vi "HXG2_PGLY-Props_R2.vi"(8 "error in (no error)":errorcluster, 9 "Temp Flowmeter (°F)":dbl, 10 "Rho PGLY Sensor(lbm/ft³)":dbl, 11 "PGLY Avg (°F)":dbl) -> (0 "error out":errorcluster, 1 "Concent":dbl, 2 "mu (lbm/ft*s)":dbl, 3 "Cp (BTU/lbm°F)":dbl, 4 "Density (lbm/ft³)":dbl)   [LabVIEW 2012]
uses:
  <vilib>/gmath/NI_Gmath.lvlib
panel:
  out "appended array":dbl[](array[numeric])
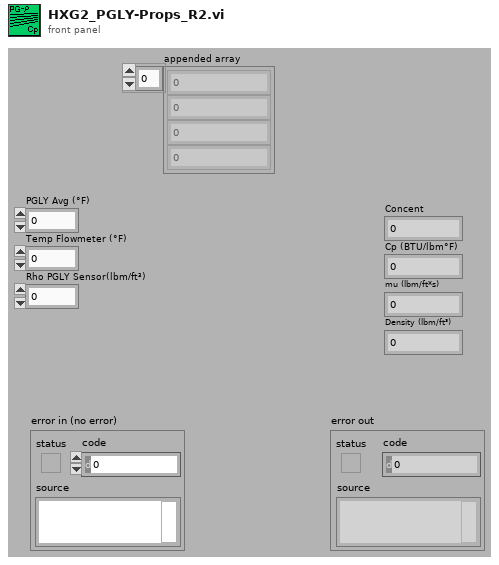
[diagram p1: front panel]
types:
  T1 = cluster{"[0]":dbl, "[1]":dbl, "[2]":dbl, "[3]":dbl}
  T2 = cluster{"[0]":dbl, "[1]":dbl, "[2]":dbl, "[3]":dbl, "[4]":dbl, "[5]":dbl, "[6]":dbl}
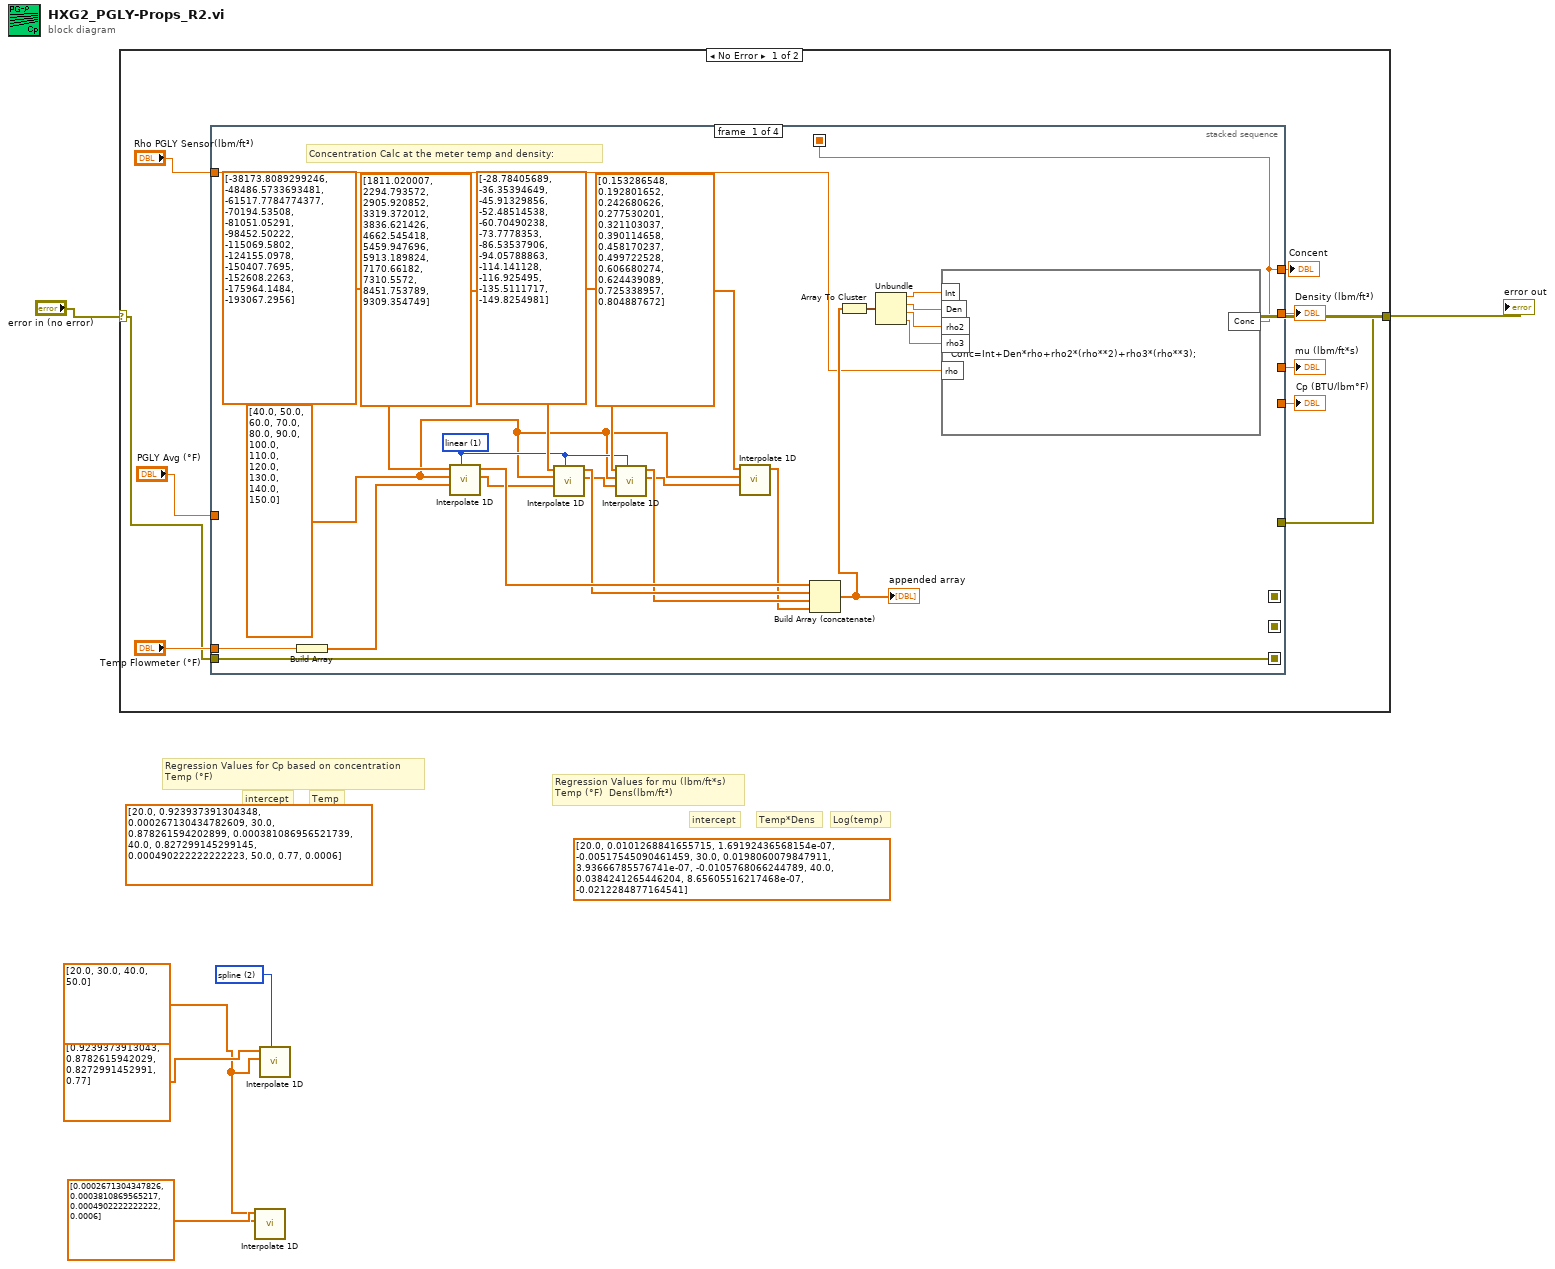
[diagram p0: block diagram]
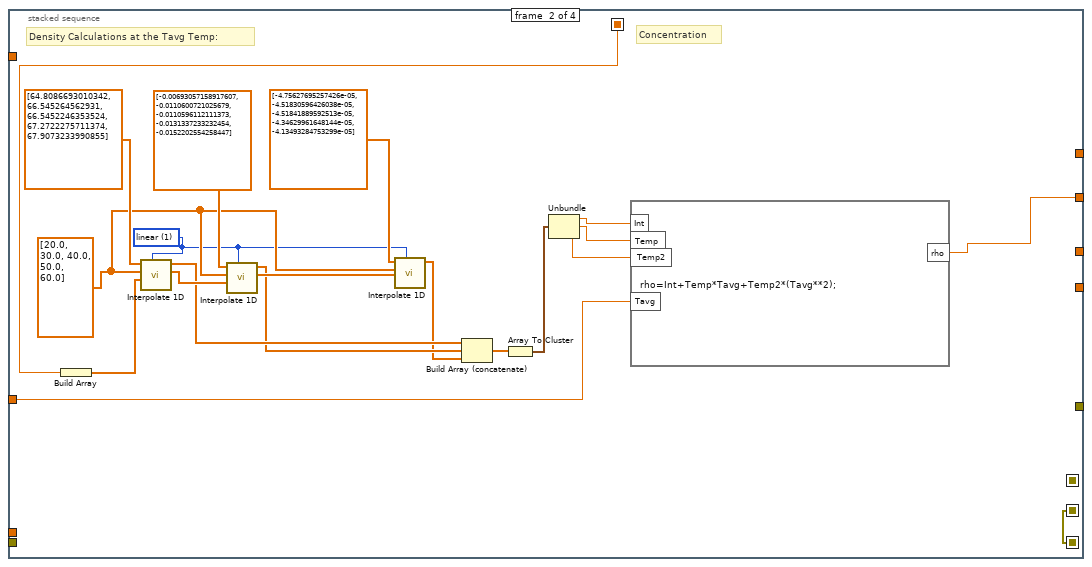
[diagram p2: hidden frame]
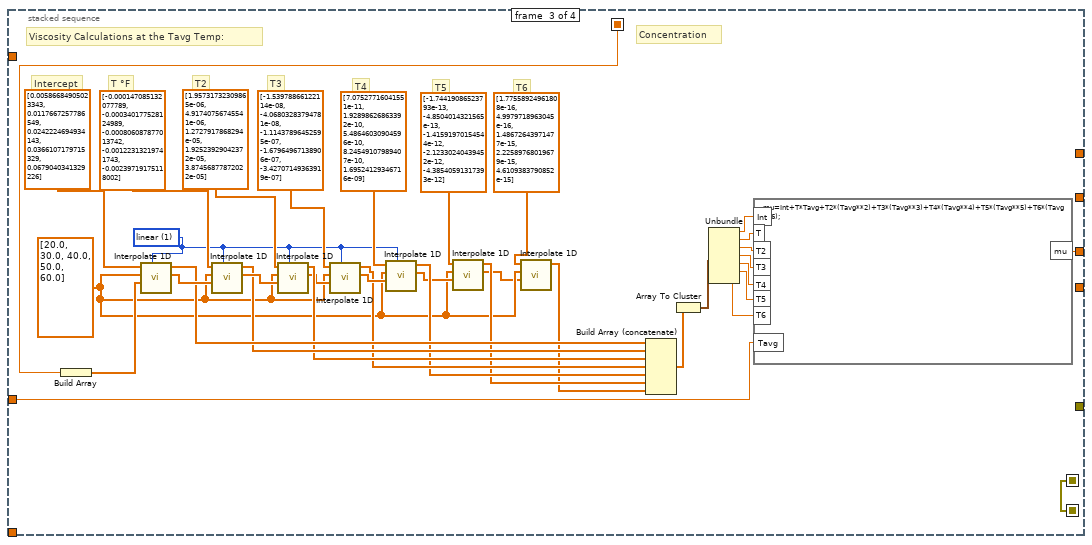
[diagram p3: hidden frame]
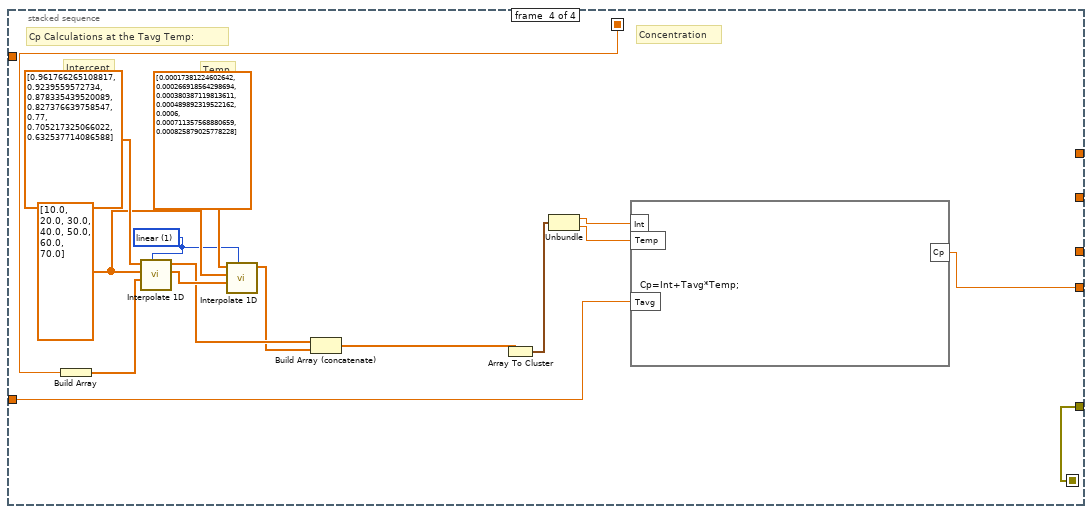
[diagram p4: hidden frame]
diagram:
  (unwired) dbl[][] [[20.0, 0.0101268841655715, 1.69192436568154e-07, -0.00517545090461459], [30.0, 0.0198060079847911, 3.93666785576741e-07, -0.0105768066244789], [40.0, 0.0384241265446204, 8.65605516217468e-07, -0.0212284877164541]]
  w4 = 2 items=["nearest", "linear", "spline", "cubic Hermite", "Lagrange"] ("method")
  w1 = dbl[] [20.0, 30.0, 40.0, 50.0] ("array")
  (unwired) dbl[][] [[20.0, 0.923937391304348, 0.000267130434782609], [30.0, 0.878261594202899, 0.000381086956521739], [40.0, 0.827299145299145, 0.000490222222222223], [50.0, 0.77, 0.0006]] ("array")
  # "Temp"
  # "intercept"
  # "Log(temp)"
  # "Temp*Dens"
  # "intercept"
  # "Regression Values for mu (lbm/ft*s)\nTemp (°F)  Dens(lbm/ft³)"
  # "Regression Values for Cp based on concentration\nTemp (°F)"
  n1 = case shown="No Error" "error in (no error)" {
    selector: "error in (no error)" -> [w12 w112]
    tunnel: [w7 w112] -> w5
    frame No Error {
      n2 = stacked-sequence {
        seq-local: [w17 _ _ _] -> [_ w43 _ _]
        seq-local: [w16 _ _ _] -> [_ w42 w82 w100]
        seq-local: [_ w43 _ _] -> [_ _ w79 _]
        seq-local: [_ _ w79 _] -> [_ _ _ w96]
        tunnel: "Temp Flowmeter (°F)" -> [w19 _ _ _]
        tunnel: "Rho PGLY Sensor(lbm/ft³)" -> [w18 _ _ _]
        tunnel: [w16 _ _ _] -> w13
        tunnel: w12 -> [w17 _ _ _]
        tunnel: [_ w44 _ _] -> w11
        tunnel: "PGLY Avg (°F)" -> [_ w40 w80 w98]
        tunnel: [_ _ w78 _] -> w9
        tunnel: [_ _ _ w97] -> w8
        tunnel: [_ _ _ w96] -> w7
        frame #0 {
          w31 = 1 items=["nearest", "linear", "spline", "cubic Hermite", "Lagrange"] ("method")
          w27 = dbl[] [40.0, 50.0, 60.0, 70.0, 80.0, 90.0, 100.0, 110.0, 120.0, 130.0, 140.0, 150.0]
          # "Concentration Calc at the meter temp and density:"
          n3 = Build Array(w19) -> (w38:dbl[])
          n4 = call <vilib>:"Interpolate 1D.vi"("method"=w31, "xi"=w38, "X"=w27, "Y"=dbl[] [-38173.8089299246, -48486.5733693481, -61517.7784774377, -70194.53508, -81051.05291, -98452.50222, -115069.5802, -124155.0978, -150407.7695, -152608.2263, -175964.1484, -193067.2956]) -> ("xi used"=w35:dbl[], "yi"=w37:dbl[])  [unwired: 5 in, 1 out]
          n5 = call <vilib>:"Interpolate 1D.vi"("method"=w31, "xi"=w35, "X"=w27, "Y"=dbl[] [1811.020007, 2294.793572, 2905.920852, 3319.372012, 3836.621426, 4662.545418, 5459.947696, 5913.189824, 7170.66182, 7310.5572, 8451.753789, 9309.354749]) -> ("xi used"=w33:dbl[], "yi"=w34:dbl[])  [unwired: 5 in, 1 out]
          n6 = call <vilib>:"Interpolate 1D.vi"("method"=w31, "xi"=w33, "X"=w27, "Y"=dbl[] [-28.78405689, -36.35394649, -45.91329856, -52.48514538, -60.70490238, -73.7778353, -86.53537906, -94.05788863, -114.141128, -116.925495, -135.5111717, -149.8254981]) -> ("xi used"=w29:dbl[], "yi"=w30:dbl[])  [unwired: 5 in, 1 out]
          n7 = call <vilib>:"Interpolate 1D.vi"("xi"=w29, "X"=w27, "Y"=dbl[] [0.153286548, 0.192801652, 0.242680626, 0.277530201, 0.321103037, 0.390114658, 0.458170237, 0.499722528, 0.606680274, 0.624439089, 0.725338957, 0.804887672]) -> ("yi"=w26:dbl[])  [unwired: 6 in, 2 out]
          n8 = Build Array (concatenate)(w37, w34, w30, w26) -> (w25:dbl[])
          "appended array" <- w25
          n9 = Array To Cluster(array=w25) -> (cluster=w24:T1)
          n10 = Unbundle(w24) -> ("[0]"=w23:dbl, "[1]"=w22:dbl, "[2]"=w21:dbl, "[3]"=w20:dbl)
          n11 = formula code="Conc=Int+Den*rho+rho2*(rho**2)+rho3*(rho**3);"("Int"=w23, "Den"=w22, "rho2"=w21, "rho3"=w20, "rho"=w18) -> ("Conc"=w16:dbl)
        }
        frame #1 {
          w53 = 1 items=["nearest", "linear", "spline", "cubic Hermite", "Lagrange"] ("method")
          w54 = dbl[] [20.0, 30.0, 40.0, 50.0, 60.0]
          # "Density Calculations at the Tavg Temp:"
          # "Concentration"
          n12 = Build Array(w42) -> (w41:dbl[])
          n13 = call <vilib>:"Interpolate 1D.vi"("method"=w53, "xi"=w41, "X"=w54, "Y"=dbl[] [64.8086693010342, 66.545264562931, 66.5452246353524, 67.2722275711374, 67.9073233990855]) -> ("xi used"=w58:dbl[], "yi"=w52:dbl[])  [unwired: 5 in, 1 out]
          n14 = call <vilib>:"Interpolate 1D.vi"("method"=w53, "xi"=w58, "X"=w54, "Y"=dbl[] [-0.00693057158917607, -0.0110600721025679, -0.0110596112111373, -0.0131337233232454, -0.0152202554258447]) -> ("xi used"=w55:dbl[], "yi"=w51:dbl[])  [unwired: 5 in, 1 out]
          n15 = call <vilib>:"Interpolate 1D.vi"("method"=w53, "xi"=w55, "X"=w54, "Y"=dbl[] [-4.75627695257426e-05, -4.51830596426038e-05, -4.51841889592513e-05, -4.34629961648144e-05, -4.13493284753299e-05]) -> ("yi"=w50:dbl[])  [unwired: 5 in, 2 out]
          n16 = Build Array (concatenate)(w52, w51, w50) -> (w49:dbl[])
          n17 = Array To Cluster(array=w49) -> (cluster=w48:cluster{"[0]":dbl, "[1]":dbl, "[2]":dbl})
          n18 = Unbundle(w48) -> ("[0]"=w47:dbl, "[1]"=w46:dbl, "[2]"=w45:dbl)
          n19 = formula code="rho=Int+Temp*Tavg+Temp2*(Tavg**2);"("Int"=w47, "Temp"=w46, "Temp2"=w45, "Tavg"=w40) -> ("rho"=w44:dbl)
        }
        frame #2 {
          w72 = 1 items=["nearest", "linear", "spline", "cubic Hermite", "Lagrange"] ("method")
          w62 = dbl[] [20.0, 30.0, 40.0, 50.0, 60.0]
          # "T6"
          # "T5"
          # "T4"
          # "T3"
          # "T2"
          # "T °F"
          # "Intercept"
          # "Viscosity Calculations at the Tavg Temp:"
          # "Concentration"
          n20 = Build Array(w82) -> (w81:dbl[])
          n21 = call <vilib>:"Interpolate 1D.vi"("method"=w72, "xi"=w81, "X"=w62, "Y"=dbl[] [0.00586684905023343, 0.0117667257786549, 0.0242224694934143, 0.0366107179715329, 0.0679040341329226]) -> ("xi used"=w94:dbl[], "yi"=w90:dbl[])  [unwired: 5 in, 1 out]
          n22 = call <vilib>:"Interpolate 1D.vi"("method"=w72, "xi"=w94, "X"=w62, "Y"=dbl[] [-0.000147085132077789, -0.000340177528124989, -0.000806087877013742, -0.00122313219741743, -0.00239719175118002]) -> ("xi used"=w91:dbl[], "yi"=w89:dbl[])  [unwired: 5 in, 1 out]
          n23 = call <vilib>:"Interpolate 1D.vi"("method"=w72, "xi"=w91, "X"=w62, "Y"=dbl[] [1.95731732309865e-06, 4.91740756745541e-06, 1.2727917868294e-05, 1.92523929042372e-05, 3.87456877872022e-05]) -> ("xi used"=w77:dbl[], "yi"=w88:dbl[])  [unwired: 5 in, 1 out]
          n24 = call <vilib>:"Interpolate 1D.vi"("method"=w72, "xi"=w77, "X"=w62, "Y"=dbl[] [-1.53978866122114e-08, -4.06803283794781e-08, -1.11437896452595e-07, -1.67964967138906e-07, -3.42707149363919e-07]) -> ("xi used"=w74:dbl[], "yi"=w73:dbl[])  [unwired: 5 in, 1 out]
          n25 = call <vilib>:"Interpolate 1D.vi"("method"=w72, "xi"=w74, "X"=w62, "Y"=dbl[] [7.07527716041551e-11, 1.92898626863392e-10, 5.48646030904596e-10, 8.24549107989407e-10, 1.69524129346716e-09]) -> ("xi used"=w68:dbl[], "yi"=w69:dbl[])  [unwired: 5 in, 1 out]
          n26 = call <vilib>:"Interpolate 1D.vi"("xi"=w68, "X"=w62, "Y"=dbl[] [-1.74419086523793e-13, -4.8504014321565e-13, -1.41591970154544e-12, -2.12330240439452e-12, -4.38540591317393e-12]) -> ("xi used"=w60:dbl[], "yi"=w67:dbl[])  [unwired: 6 in, 1 out]
          n27 = call <vilib>:"Interpolate 1D.vi"("xi"=w60, "X"=w62, "Y"=dbl[] [1.77558924961808e-16, 4.9979718963045e-16, 1.48672643971477e-15, 2.22589768019679e-15, 4.6109383790852e-15]) -> ("yi"=w61:dbl[])  [unwired: 6 in, 2 out]
          n28 = Build Array (concatenate)(w90, w89, w88, w73, w69, w67, w61) -> (w87:dbl[])
          n29 = Array To Cluster(array=w87) -> (cluster=w86:T2)
          n30 = Unbundle(w86) -> ("[0]"=w85:dbl, "[1]"=w84:dbl, "[2]"=w83:dbl, "[3]"=w71:dbl, "[4]"=w70:dbl, "[5]"=w66:dbl, "[6]"=w65:dbl)
          n31 = formula code="mu=Int+T*Tavg+T2*(Tavg**2)+T3*(Tavg**3)+T4*(Tavg**4)+T5*(Tavg**5)+T6*(Tavg**6);"("Int"=w85, "T"=w84, "T2"=w83, "Tavg"=w80, "T3"=w71, "T4"=w70, "T5"=w66, "T6"=w65) -> ("mu"=w78:dbl)
        }
        frame #3 {
          w107 = 1 items=["nearest", "linear", "spline", "cubic Hermite", "Lagrange"] ("method")
          w108 = dbl[] [10.0, 20.0, 30.0, 40.0, 50.0, 60.0, 70.0]
          # "Temp"
          # "Intercept"
          # "Cp Calculations at the Tavg Temp:"
          # "Concentration"
          n32 = Build Array(w100) -> (w99:dbl[])
          n33 = call <vilib>:"Interpolate 1D.vi"("method"=w107, "xi"=w99, "X"=w108, "Y"=dbl[] [0.961766265108817, 0.9239559572734, 0.878335439520089, 0.827376639758547, 0.77, 0.705217325066022, 0.632537714086588]) -> ("xi used"=w110:dbl[], "yi"=w106:dbl[])  [unwired: 5 in, 1 out]
          n34 = call <vilib>:"Interpolate 1D.vi"("method"=w107, "xi"=w110, "X"=w108, "Y"=dbl[] [0.00017381224602642, 0.000266918564298694, 0.000380387119813611, 0.000489892319522162, 0.0006, 0.000711357568880659, 0.000825879025778228]) -> ("yi"=w105:dbl[])  [unwired: 5 in, 2 out]
          n35 = Build Array (concatenate)(w106, w105) -> (w104:dbl[])
          n36 = Array To Cluster(array=w104) -> (cluster=w103:cluster{"[0]":dbl, "[1]":dbl})
          n37 = Unbundle(w103) -> ("[0]"=w102:dbl, "[1]"=w101:dbl)
          n38 = formula code="Cp=Int+Tavg*Temp;"("Int"=w102, "Temp"=w101, "Tavg"=w98) -> ("Cp"=w97:dbl)
        }
      }
      "Concent" <- w13
      "Density (lbm/ft³)" <- w11
      "mu (lbm/ft*s)" <- w9
      "Cp (BTU/lbm°F)" <- w8
    }
    frame Error {
    }
  }
  "error out" <- w5
  n39 = call <vilib>:"Interpolate 1D.vi"("X"=w1, "Y"=dbl[] [0.0002671304347826, 0.0003810869565217, 0.0004902222222222, 0.0006] ("array")) -> ()  [unwired: 7 in, 3 out]
  n40 = call <vilib>:"Interpolate 1D.vi"("method"=w4, "X"=w1, "Y"=dbl[] [0.9239373913043, 0.8782615942029, 0.8272991452991, 0.77] ("array")) -> ()  [unwired: 6 in, 3 out]
